vi "(Sub VI) Parse move C.vi"(11 "data":string) -> (2 "Motion parameters":T2, 3 "Position C":T1 {"X" format="%.4f"; "Y" format="%.4f"; "Z" format="%.4f"; "Rx" format="%.4f"; "Ry" format="%.4f"; "Rz" format="%.4f"})   [LabVIEW 2022 SP3]
uses:
  <vilib>/ImagingLab/Denso Robotics Library/_Private/Controls/drl_Interpolation.ctl
  <vilib>/ImagingLab/Denso Robotics Library/DensoRoboticsLibrary.lvlib
  <vilib>/ImagingLab/Denso Robotics Library/_Private/Controls/drl_Pass motion.ctl
  <vilib>/ImagingLab/Denso Robotics Library/_Private/Controls/drl_Move option.ctl
  <vilib>/ImagingLab/Denso Robotics Library/_Private/Controls/drl_Motion parameters.ctl
  <vilib>/ImagingLab/Denso Robotics Library/_Private/Controls/drl_Robot Coordinates.ctl
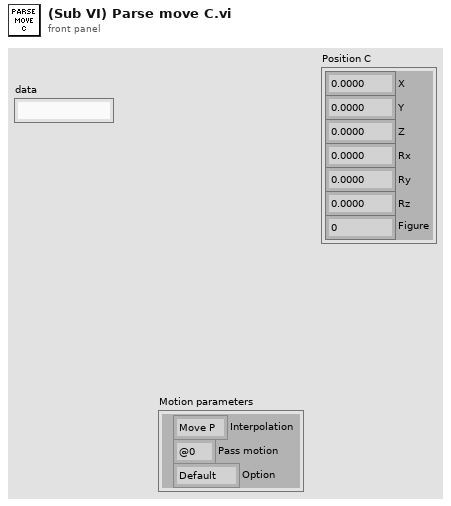
[diagram p1: front panel]
types:
  T1 = typedef "DensoRoboticsLibrary.lvlib/drl_Robot Coordinates.ctl" = cluster{"X":dbl, "Y":dbl, "Z":dbl, "Rx":dbl, "Ry":dbl, "Rz":dbl, "Figure":dbl}
  T2 = typedef "DensoRoboticsLibrary.lvlib/drl_Motion parameters.ctl" = cluster{"Interpolation":T3, "Pass motion":T4, "Option":T5}
  T3 = typedef "DensoRoboticsLibrary.lvlib/drl_Interpolation.ctl" = enum16{"Move P", "Move L"}
  T4 = typedef "DensoRoboticsLibrary.lvlib/drl_Pass motion.ctl" = enum16{"@0", "@P", "@E"}
  T5 = typedef "DensoRoboticsLibrary.lvlib/drl_Move option.ctl" = enum16{"Default", "Next"}
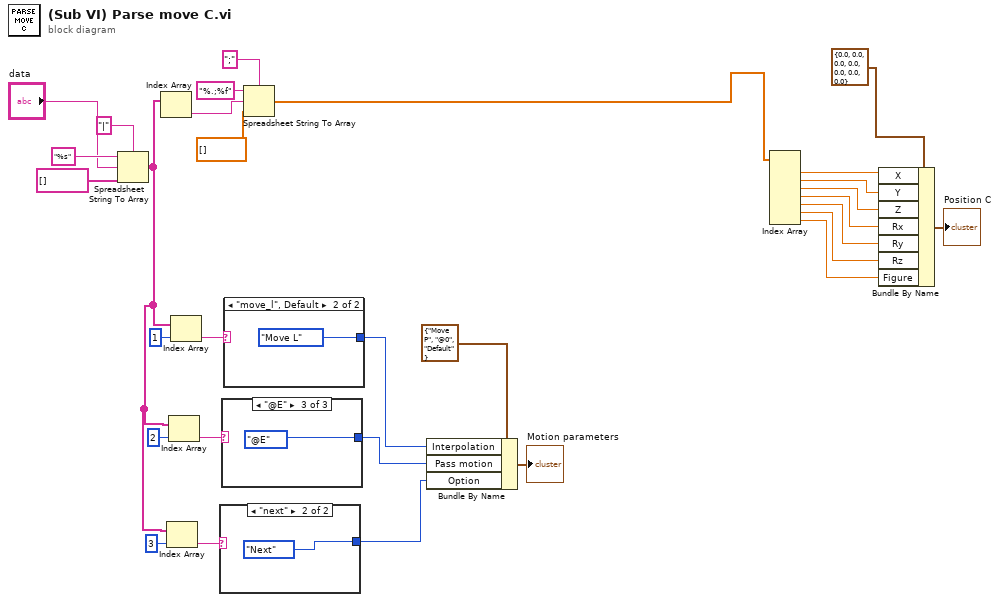
[diagram p0: block diagram]
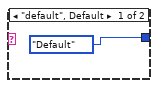
[diagram p2: hidden frame]
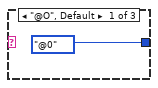
[diagram p3: hidden frame]
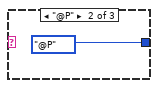
[diagram p4: hidden frame]
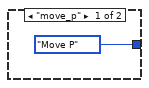
[diagram p5: hidden frame]
diagram:
  n1 = Spreadsheet String To Array(delimiter (Tab)="|", format string="%s", spreadsheet string="data", array type (2D Dbl)=string[] []) -> (array=w25:string[])
  n2 = Index Array(array=w25) -> (element=w18:string)  [unwired: 1 in]
  n3 = Index Array(array=w25, index=3) -> (element=w23:string)
  n4 = Index Array(array=w25, index=2) -> (element=w22:string)
  n5 = Index Array(array=w25, index=1) -> (element=w19:string)
  n6 = case shown="\"next\"" w23 {
    tunnel: [drl_Move_option."Default" ("Option") drl_Move_option."Next" ("Option")] -> w28
    frame "default", Default {
    }
    frame "next" {
    }
  }
  n7 = case shown="\"@E\"" w22 {
    tunnel: [drl_Pass_motion."@0" ("Pass motion") drl_Pass_motion."@P" ("Pass motion") drl_Pass_motion."@E" ("Pass motion")] -> w27
    frame "@O", Default {
    }
    frame "@P" {
    }
    frame "@E" {
    }
  }
  n8 = case shown="\"move_l\", Default" w19 {
    tunnel: [drl_Interpolation."Move P" ("Interpolation") drl_Interpolation."Move L" ("Interpolation")] -> w26
    frame "move_p" {
    }
    frame "move_l", Default {
    }
  }
  n9 = Spreadsheet String To Array(delimiter (Tab)=";", format string="%.;%f", spreadsheet string=w18, array type (2D Dbl)=dbl[] []) -> (array=w1:dbl[])
  n10 = Bundle By Name(cluster=T2 {"Interpolation"=enum."Move P", "Pass motion"=enum."@0", "Option"=enum."Default"} ("motion parameters"), "Interpolation"=w26, "Pass motion"=w27, "Option"=w28) -> (→"Motion parameters":T2)
  n11 = Index Array(array=w1) -> (element #1=w10:dbl, element #2=w9:dbl, element #3=w8:dbl, element #4=w7:dbl, element #5=w6:dbl, element #6=w5:dbl, element #7=w3:dbl)  [unwired: 7 in]
  n12 = Bundle By Name(cluster=T1 {"X"=0.0, "Y"=0.0, "Z"=0.0, "Rx"=0.0, "Ry"=0.0, "Rz"=0.0, "Figure"=0.0} ("robot coordinates"), "X"=w10, "Y"=w9, "Z"=w8, "Rx"=w7, "Ry"=w6, "Rz"=w5, "Figure"=w3) -> (→"Position C":T1)
